vi "Create Status Channels.vi"(8 "error in (no error)":errorcluster, 11 "Output Sequencer in":refnum<class "Output Sequencer.lvclass">) -> (0 "error out":errorcluster, 3 "Output Sequencer out":refnum<class "Output Sequencer.lvclass">)   [LabVIEW 2024, in "Output Sequencer.lvlib" / "Output Sequencer.lvclass"]
uses:
  Output Sequencer.lvclass
  <vilib>/FlexLogger/SDK/PluginSDK.lvlibp/PEFClasses/SDK/Channel/Data Type_v2.ctl
  <vilib>/FlexLogger/SDK/PluginSDK.lvlibp/PEFClasses/SDK/Producer Channel/Producer Channel.lvclass
  C:/Program Files/National Instruments/LabVIEW 2024/vi.lib/FlexLogger/SDK/PluginSDK.lvlibp/PEFClasses/SDK/Channel/Channel.lvclass
  Globals/Global Strings.vi
  <vilib>/FlexLogger/SDK/PluginSDK.lvlibp/PEFClasses/SDK/Producer Channel/Create Producer Channel_v2.vi
  <vilib>/FlexLogger/SDK/PluginSDK.lvlibp/PEFClasses/SDK/Plugin/Plugin.lvclass
  <vilib>/FlexLogger/SDK/PluginSDK.lvlibp
  <vilib>/FlexLogger/SDK/PluginSDK.lvlibp/PEFClasses/SDK/Channel/Channel.lvclass
  C:/Program Files/National Instruments/LabVIEW 2024/vi.lib/FlexLogger/SDK/PluginSDK.lvlibp/PEFClasses/SDK/Plugin/Plugin.lvclass
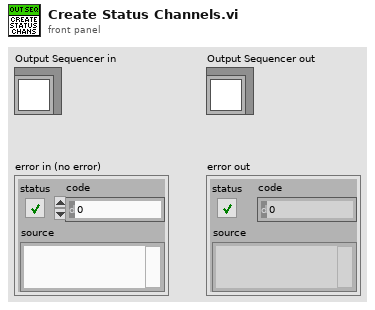
[diagram p1: front panel]
types:
  T1 = typedef "PluginSDK.lvlibp/Channel.lvclass/Data Type_v2.ctl" = u16
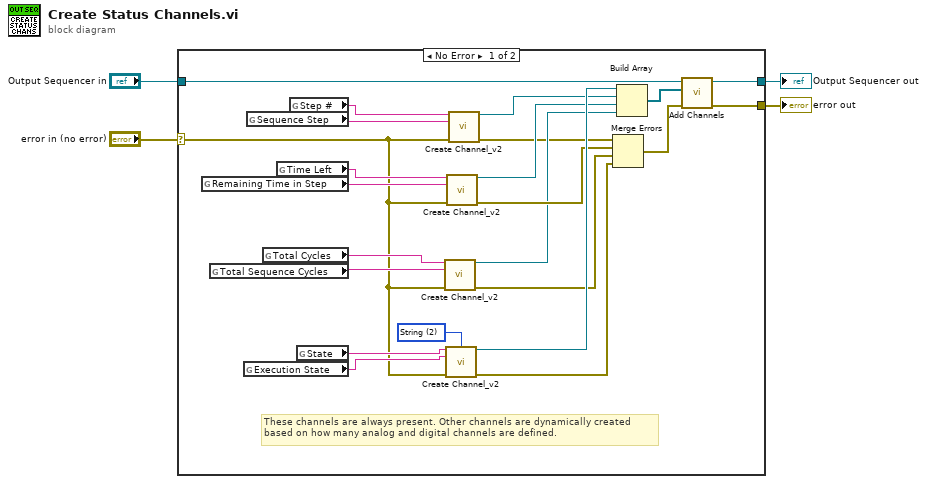
[diagram p0: block diagram]
diagram:
  n1 = case shown="No Error" "error in (no error)" {
    selector: "error in (no error)" -> [w5 w28]
    tunnel: "Output Sequencer in" -> [w27 w29]
    tunnel: [w21 w29] -> w3
    tunnel: [w20 w28] -> w2
    frame No Error {
      w22 = T1 2 items=["Wfm (DBL)", "Wfm (Digital)", "String"] ("Data Type")
      # "These channels are always present. Other channels are dynamically created\nbased on how many analog and digital channels are defined."
      n2 = global read "Global Strings.vi" "Remaining Time in Step"() -> (w16:string)
      n3 = global read "Global Strings.vi" "Total Sequence Cycles"() -> (w18:string)
      n4 = global read "Global Strings.vi" "Execution State"() -> (w25:string)
      n5 = global read "Global Strings.vi" "Sequence Step"() -> (w14:string)
      n6 = global read "Global Strings.vi" "Total Cycles"() -> (w19:string)
      n7 = global read "Global Strings.vi" "Time Left"() -> (w17:string)
      n8 = global read "Global Strings.vi" "Step #"() -> (w15:string)
      n9 = global read "Global Strings.vi" "State"() -> (w24:string)
      n10 = call-poly <vilib>:"Create Channel_v2.vi"("Unique Channel Identifier"=w19, "Default Channel Name"=w18, "error in (no error)"=w5) -> ("Producer Channel"=w11:refnum<class "Producer Channel.lvclass">, "error out"=w13:errorcluster)  [unwired: 11 in]
      n11 = call-poly <vilib>:"Create Channel_v2.vi"("Unique Channel Identifier"=w24, "Data Type"=w22, "Default Channel Name"=w25, "error in (no error)"=w5) -> ("Producer Channel"=w23:refnum<class "Producer Channel.lvclass">, "error out"=w26:errorcluster)  [unwired: 10 in]
      n12 = call-poly <vilib>:"Create Channel_v2.vi"("Unique Channel Identifier"=w17, "Default Channel Name"=w16, "error in (no error)"=w5) -> ("Producer Channel"=w10:refnum<class "Producer Channel.lvclass">, "error out"=w12:errorcluster)  [unwired: 11 in]
      n13 = call-poly <vilib>:"Create Channel_v2.vi"("Unique Channel Identifier"=w15, "Default Channel Name"=w14, "error in (no error)"=w5) -> ("Producer Channel"=w9:refnum<class "Producer Channel.lvclass">, "error out"=w8:errorcluster)  [unwired: 11 in]
      n14 = Merge Errors(w8, w12, w13, w26) -> (w7:errorcluster)
      n15 = Build Array(w23, w9, w10, w11) -> (w6:refnum<class "Producer Channel.lvclass">[])
      n16 = call <vilib>:"Add Channels.vi"("error in (no error)"=w7, "Channels"=w6, "Plugin in"=w27) -> ("error out"=w20:errorcluster, "Plugin out"=w21:refnum<class "Output Sequencer.lvclass">)  [unwired: 7 in]
    }
    frame Error {
    }
  }
  "Output Sequencer out" <- w3
  "error out" <- w2
